vi "Y[i]=X[i-n].vi"(2 "shifts: n":i32, 3 "Input Array":dbl[](array[numeric])) -> (0 "error":i32, 1 "Shifted Array":dbl[](array[numeric]))   [LabVIEW 2020, in "NI_AALPro.lvlib"]
doc: "Shifts the elements in the <B>Input Array</B> by the specified number of <B>shifts: n</B>."
uses:
  <vilib>/Analysis/NI_AALPro.lvlib
panel:
  # "Y[i]=X[i-n]"
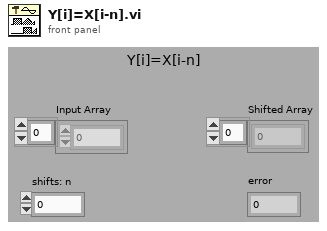
[diagram p1: front panel]
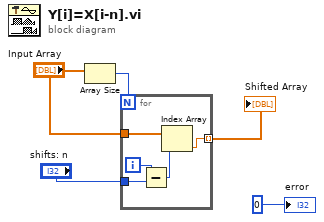
[diagram p0: block diagram]
diagram:
  n1 = Array Size(array="Input Array") -> (size(s)=w2:i32)
  n2 = for {
    N: w2 -> [_]
    tunnel: "shifts: n" -> [w9]
    tunnel: "Input Array" -> [w7]
    tunnel: [w6] -> w3 mode=indexing
    i -> [w10]
    n3 = Subtract(x=w10, y=w9) -> (x-y=w8:i32)
    n4 = Index Array(array=w7, index=w8) -> (element=w6:dbl)
  }
  "Shifted Array" <- w3
  "error" <- 0
